vi "RFU_Rsrc.vi"(7 "RFU":T1, 8 "error in (no error)":errorcluster) -> (0 "error out":errorcluster, 2 "K7_1":refnum<visa-resource-name>, 3 "K7_0":refnum<visa-resource-name>)   [LabVIEW 2018]
uses:
  Types/RFU.ctl
  <vilib>/Utility/config.llb/Read Key (String).vi
  <vilib>/Utility/config.llb/NI_LVConfig.lvlib
panel:
  out "K7_1":string
  out "K7_0":string
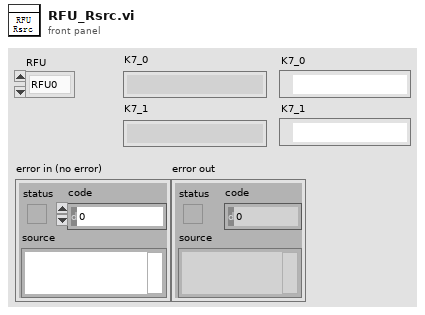
[diagram p1: front panel]
types:
  T1 = typedef "RFU.ctl" = enum8{"RFU0", "RFU1", "RFU2", "RFU3", "RFU4"}
  T2 = typedef "NI_LVConfig.lvlib/Config Data RefNum.ctl" = refnum<k1>
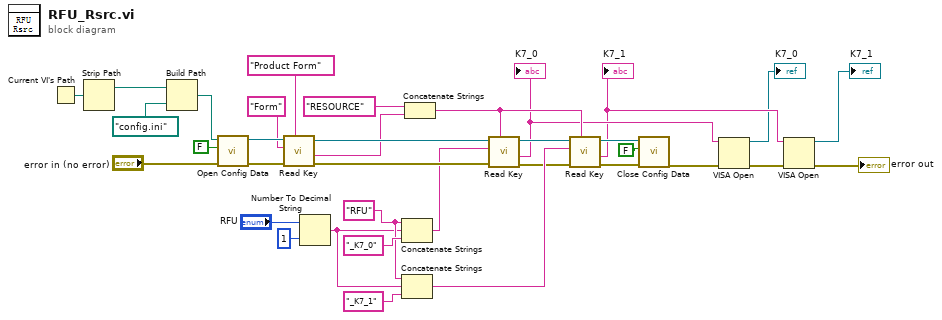
[diagram p0: block diagram]
diagram:
  w21 = "RFU" ("string")
  n1 = Current VI's Path() -> (path=w9:path)
  n2 = Strip Path(path=w9) -> (stripped path=w8:path)  [unwired: 1 out]
  n3 = Build Path(base path=w8, name or relative path=path "config.ini" ("configuration file path")) -> (appended path=w10:path)
  n4 = call <vilib>:"Open Config Data.vi"("error in (no error)"="error in (no error)", "create file if necessary (T)"=FALSE, "configuration file path"=w10) -> ("error out"=w32:errorcluster, "refnum"=w33:T2)  [unwired: 6 in, 1 out]
  n5 = call-poly <vilib>:"Read Key.vi"("section"="Product Form", "error in (no error)"=w32, "key"="Form", "refnum"=w33) -> ("error out"=w28:errorcluster, "value"=w26:string, "refnum out"=w29:T2)  [unwired: 4 in, 1 out]
  n6 = Number To Decimal String(number="RFU", width (-)=i16 1) -> (decimal integer string=w20:string)
  n7 = Concatenate Strings(w21, w20, "_K7_0" ("string")) -> (w19:string)
  n8 = Concatenate Strings(w21, w20, "_K7_1" ("string")) -> (w16:string)
  n9 = Concatenate Strings("RESOURCE" ("string"), w26) -> (w17:string)
  n10 = call-poly <vilib>:"Read Key.vi"("section"=w17, "error in (no error)"=w28, "key"=w19, "refnum"=w29) -> ("error out"=w15:errorcluster, "value"=w6:string, "refnum out"=w18:T2)  [unwired: 4 in, 1 out]
  "K7_0" <- w6
  n11 = call-poly <vilib>:"Read Key.vi"("section"=w17, "error in (no error)"=w15, "key"=w16, "refnum"=w18) -> ("error out"=w14:errorcluster, "value"=w4:string, "refnum out"=w13:T2)  [unwired: 4 in, 1 out]
  "K7_1" <- w4
  n12 = call <vilib>:"Close Config Data.vi"("error in (no error)"=w14, "write file if changed (T)"=FALSE, "refnum"=w13) -> ("error out"=w7:errorcluster)  [unwired: 7 in, 1 out]
  n13 = VISA Open(error in (no error)=w7, VISA resource name=w6) -> (VISA resource name=→"K7_0":refnum<visa-resource-name>, error out=w5:errorcluster)  [unwired: 3 in]
  n14 = VISA Open(error in (no error)=w5, VISA resource name=w4) -> (VISA resource name=→"K7_1":refnum<visa-resource-name>, error out=→"error out":errorcluster)  [unwired: 3 in]
